vi "Globals Summary.vi"() -> ()   [LabVIEW 2016, in "Transport.lvclass"]
uses:
  Transport.lvclass
  <userlib>/LevyLab/Krohn Hite 7008/SMOs/KH7008/typedefs/KH_control_array.ctl
  <userlib>/LevyLab/Krohn Hite 7008/SMOs/KH7008/typedefs/KH_control.ctl
  <userlib>/LevyLab/Krohn Hite 7008/SMOs/KH7008/typedefs/Channel-Enum.ctl
  <userlib>/LevyLab/Krohn Hite 7008/SMOs/KH7008/typedefs/Gain-Enum.ctl
  <userlib>/LevyLab/Krohn Hite 7008/SMOs/KH7008/typedefs/Shunt-Enum.ctl
  <userlib>/LevyLab/Krohn Hite 7008/SMOs/KH7008/typedefs/Input Configuration-Enum.ctl
  <userlib>/LevyLab/Lockin-Multichannel/Typedefs/AI.config-array.ctl
  <userlib>/LevyLab/Lockin-Multichannel/Typedefs/AI.config-cluster.ctl
  <userlib>/LevyLab/Lockin-Multichannel/Typedefs/AI.coupling-enum.ctl
  <userlib>/LevyLab/Lockin-Multichannel/Typedefs/446xAI-enum.ctl
  <userlib>/LevyLab/Lockin-Multichannel/Typedefs/AO-cluster.ctl
  <userlib>/LevyLab/Lockin-Multichannel/Typedefs/AO_Amp-array.ctl
  <userlib>/LevyLab/Lockin-Multichannel/Typedefs/AO_DC-array.ctl
  <userlib>/LevyLab/Lockin-Multichannel/Typedefs/AO_f-array.ctl
  <userlib>/LevyLab/Lockin-Multichannel/Typedefs/AO_phi-array.ctl
  <userlib>/LevyLab/Lockin-Multichannel/Typedefs/Function-array.ctl
  <userlib>/LevyLab/Lockin-Multichannel/Typedefs/Function-enum.ctl
  <userlib>/LevyLab/Krohn Hite 7008/SMOs/KH7008/KH7008.lvclass
panel:
  out "filename":string="SA01234.20180713"
  out "folder":string="G:\\Team Drives\\LevyLabData/quasi-1D chiral proteins/SA01234.20180713"
  out "comments":string="SA01234.20180713\nquasi-1D chiral proteins\npatrick"
  in  "user (emum?)":string="patrick"
  in  "project":string="quasi-1D chiral proteins"
  out "device":string="SA01234.20180713"
  in  "device":string="20180713"
  in  "sample":string="SA01234"
  in  "image path":string
  in  "Channels: AO":T1={"AO amp (V)"=[0.01, 0.0, 0.0, 0.0, 0.0, 0.0, 0.0, 0.0], "AO DC (V)"=[0.0, 0.0, 0.0, 0.0, 0.0, 0.0, 0.0, 0.0], "AO f (Hz)"=[13.1, 13.0, 13.0, 13.0, 13.0, 13.0, 13.0, 13.0], "AO phi (deg)"=[0.0, 0.0, 0.0, 0.0, 0.0, 0.0, 0.0, 0.0], "function"=[enum."Sine Wave", enum."Sine Wave", enum."Sine Wave", enum."Sine Wave", enum."Sine Wave", enum."Sine Wave", enum."Sine Wave", enum."Sine Wave"]} {"AO f (Hz)" min=0.001 max=10000.0; "AO DC (V)" format="%#_6p"; "AO amp (V)" format="%#_6p"}
  in  "AI Configuration":T8=[{"AI.Coupling"=enum."GND", "AI.channels"="", "AI.Range"=enum."±0.316 V"}, {"AI.Coupling"=enum."GND", "AI.channels"="", "AI.Range"=enum."±0.316 V"}, {"AI.Coupling"=enum."GND", "AI.channels"="", "AI.Range"=enum."±0.316 V"}, {"AI.Coupling"=enum."GND", "AI.channels"="Dev2/ai0", "AI.Range"=enum."±0.316 V"}]
  in  "V4-":dbl
  in  "V4+":dbl
  in  "comments":string
  in  "folder":string
  in  "Channel Setting":T12=[{"Channel"=enum."Channel 2", "Gain"=enum."10x", "Shunt Resistor"=enum."50 Ohms", "Input Config"=enum."Differential"}, {"Channel"=enum."Channel 2", "Gain"=enum."10x", "Shunt Resistor"=enum."50 Ohms", "Input Config"=enum."Differential"}, {"Channel"=enum."Channel 2", "Gain"=enum."10x", "Shunt Resistor"=enum."50 Ohms", "Input Config"=enum."Differential"}, {"Channel"=enum."Channel 2", "Gain"=enum."10x", "Shunt Resistor"=enum."50 Ohms", "Input Config"=enum."Differential"}, {"Channel"=enum."Channel 2", "Gain"=enum."10x", "Shunt Resistor"=enum."50 Ohms", "Input Config"=enum."Differential"}, {"Channel"=enum."Channel 2", "Gain"=enum."10x", "Shunt Resistor"=enum."50 Ohms", "Input Config"=enum."Differential"}, {"Channel"=enum."Channel 2", "Gain"=enum."10x", "Shunt Resistor"=enum."50 Ohms", "Input Config"=enum."Differential"}, {"Channel"=enum."Channel 2", "Gain"=enum."10x", "Shunt Resistor"=enum."50 Ohms", "Input Config"=enum."Differential"}]
  in  "V3-":dbl
  in  "V3+":dbl
  in  "V2-":dbl
  in  "V2+":dbl
  in  "V1-":dbl
  in  "V1+":dbl
  in  "I-":dbl
  in  "I+":dbl
  in  "pickering path":string
  in  "PPMS T&B logfile":string
  in  "filename":string
  in  "folder":string
  # "Experiment stuff"
  # "\"Channel Globals\""
  # "\"ITX Globals\""
  # "I think we should have the following also:"
  # "auto created:"
  # "necessary?"
  # "necessary?"
  # "necessary?"
  # "Lockin Settings (owned by lockin package)"
  # "KH Settings (owned by KH package)"
  # "0"
  # "1"
  # "2"
  # "3"
  # "4"
  # "5"
  # "6"
  # "7"
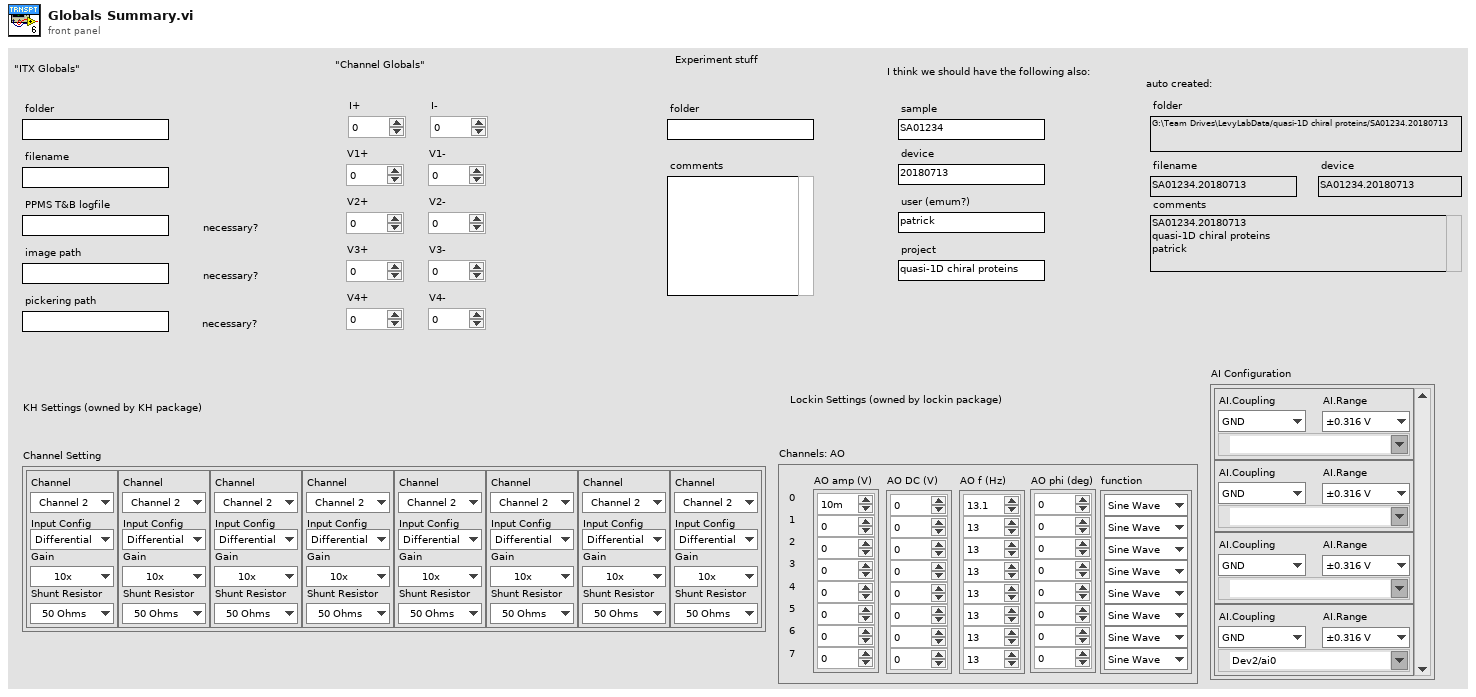
[diagram p1: front panel]
types:
  T1 = typedef "AO-cluster.ctl" = cluster{"AO amp (V)":T2, "AO DC (V)":T3, "AO f (Hz)":T4, "AO phi (deg)":T5, "function":T6}
  T2 = typedef "AO_Amp-array.ctl" = dbl[]
  T3 = typedef "AO_DC-array.ctl" = dbl[]
  T4 = typedef "AO_f-array.ctl" = dbl[]
  T5 = typedef "AO_phi-array.ctl" = dbl[]
  T6 = typedef "Function-array.ctl" = T7[]
  T7 = typedef "Function-enum.ctl" = enum16{"Sine Wave", "Triangle Wave", "Square Wave", "Sawtooth Wave"}
  T8 = typedef "AI.config-array.ctl" = T9[]
  T9 = typedef "AI.config-cluster.ctl" = cluster{"AI.Coupling":T10, "AI.channels":tag, "AI.Range":T11}
  T10 = typedef "AI.coupling-enum.ctl" = enum16{"AC", "DC", "GND"}
  T11 = typedef "446xAI-enum.ctl" = enum16{"±0.316 V", "±1.00 V", "±3.16 V", "±10.0 V", "±31.6 V", "±42.4 V"}
  T12 = typedef "KH7008.lvclass/KH_control_array.ctl" = T13[]
  T13 = typedef "KH7008.lvclass/KH_control.ctl" = cluster{"Channel":T14, "Gain":T15, "Shunt Resistor":T16, "Input Config":T17}
  T14 = typedef "KH7008.lvclass/Channel-Enum.ctl" = enum16{"Channel 1", "Channel 2", "Channel 3", "Channel 4", "Channel 5", "Channel 6", "Channel 7", "Channel 8"}
  T15 = typedef "KH7008.lvclass/Gain-Enum.ctl" = enum16{"1x", "10x", "100x", "1000x"}
  T16 = typedef "KH7008.lvclass/Shunt-Enum.ctl" = enum16{"Open", "50 Ohms", "500 Ohms", "5k Ohms", "50k Ohms"}
  T17 = typedef "KH7008.lvclass/Input Configuration-Enum.ctl" = enum16{"Ground", "SE+ (-gnd)", "SE- (+gnd)", "Differential"}
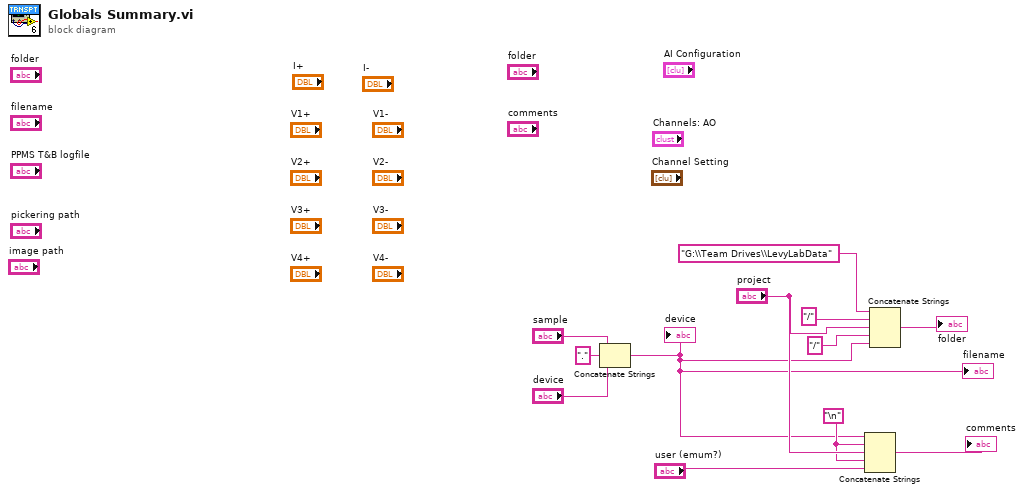
[diagram p0: block diagram]
diagram:
  w3 = "\n"
  n1 = Concatenate Strings("sample", "." ("string"), "device") -> (w1:string)
  "device" <- w1
  "filename" <- w1
  n2 = Concatenate Strings(w1, w3, "project", w3, "user (emum?)") -> (→"comments":string)
  n3 = Concatenate Strings("G:\\Team Drives\\LevyLabData" ("string"), "/" ("string"), "project", "/" ("string"), w1) -> (→"folder":string)
